vi "ContextHelp_StopPopUpTask.vi"(5 "error in (no error)":errorcluster) -> (19 "error out":errorcluster)   [LabVIEW 2016]
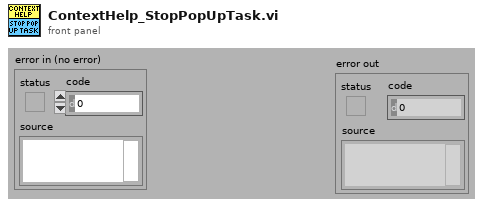
[diagram p1: front panel]
types:
  T1 = enum16{"SetPopUpEventTask", "GetStatus", "SetOpenState", "SetDialogCaller"}
  T2 = typedef "ContextHelp_EventType.ctl" = refnum<user-event>
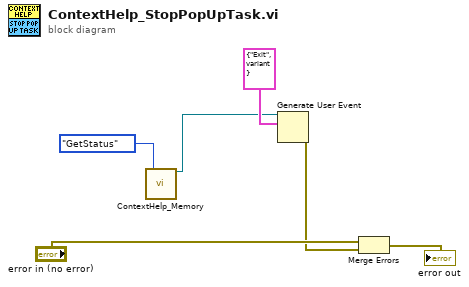
[diagram p0: block diagram]
diagram:
  n1 = call <resource>:"ContextHelp_Memory.vi"("Actio(GetStatus)n"=T1."GetStatus") -> ("PopUpTaskEventOut"=w2:T2)  [unwired: 3 in, 15 out]
  n2 = Generate User Event(user event=w2, event data cluster=cluster{"Command":string, "Data":variant} {"Command"="Exit", "Data"=variant} ("event data")) -> (error out=w4:errorcluster)  [unwired: 2 in, 1 out]
  n3 = Merge Errors("error in (no error)", w4) -> (→"error out":errorcluster)
